vi "ByteArrayToImage.vi"(0 "CameraBytes":u8[](array[numeric]), 1 "Image":T1) -> (5 "Image Out":T1)   [LabVIEW 2019]
uses:
  <vilib>/vision/Image Controls.llb/IMAQ Image.ctl
  <vilib>/vision/NI_Vision_Development_Module.lvlib
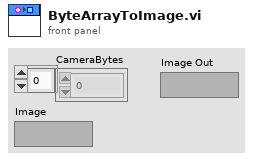
[diagram p1: front panel]
types:
  T1 = typedef "IMAQ Image.ctl" = refnum<image>
  T2 = cluster{"Red or Hue value":u8, "Green or Sat value":u8, "Blue or Luma or Val or Inten value":u8}
  T3 = cluster{"Red or Hue value":u8, "Green or Sat value":u8, "Blue or Luma or Val or Inten value":u8}[]
  T4 = cluster{"Red or Hue value":u8, "Green or Sat value":u8, "Blue or Luma or Val or Inten value":u8}[][]
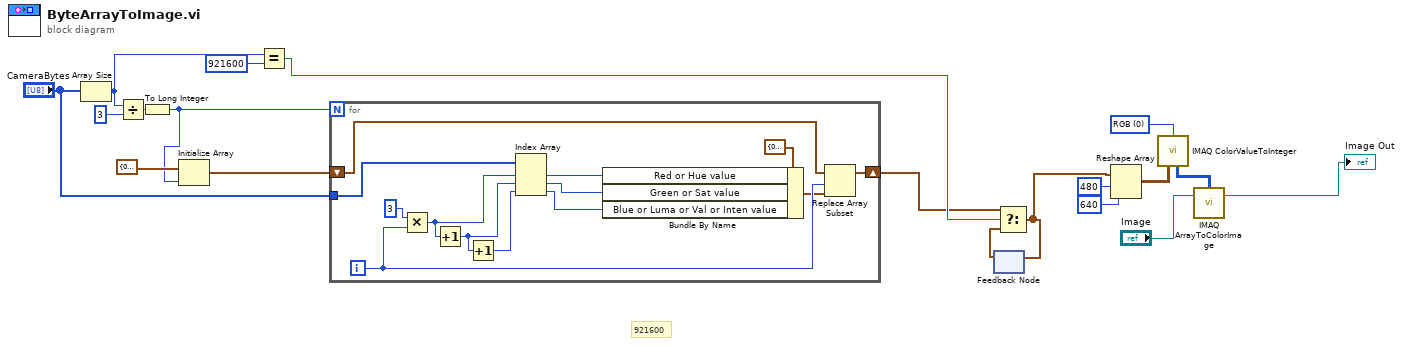
[diagram p0: block diagram]
diagram:
  w11 = u16 0 items=["RGB", "HSL", "HSV", "HSI"] ("Color Mode")
  # "921600"
  n1 = Array Size(array="CameraBytes") -> (size(s)=w1:i32)
  n2 = Divide(x=w1, y=3) -> (x/y=w17:dbl)
  n3 = To Long Integer(number=w17) -> (32bit integer=w7:i32)
  n4 = Initialize Array(T2 {"Red or Hue value"=0, "Green or Sat value"=0, "Blue or Luma or Val or Inten value"=0} ("Color Value"), w7) -> (w15:T3)
  n5 = Equal?(x=w1, y=921600) -> (x = y?=w5:bool)
  n6 = for {
    N: w7 -> [_]
    tunnel: "CameraBytes" -> [w30]
    shift-right: [w21] -> w4
    shift-left: w15 -> [w20]
    i -> [w23]
    n7 = Multiply(x=3, y=w23) -> (x*y=w26:i32)
    n8 = Increment(x=w26) -> (x+1=w25:i32)
    n9 = Increment(x=w25) -> (x+1=w24:i32)
    n10 = Index Array(array=w30, index #1=w26, index #2=w25, index #3=w24) -> (element #1=w29:u8, element #2=w28:u8, element #3=w27:u8)
    n11 = Bundle By Name(cluster=T2 {"Red or Hue value"=0, "Green or Sat value"=0, "Blue or Luma or Val or Inten value"=0} ("Color Value"), "Red or Hue value"=w29, "Green or Sat value"=w28, "Blue or Luma or Val or Inten value"=w27) -> (w22:T2)
    n12 = Replace Array Subset(array=w20, new element=w22, index=w23) -> (w21:T3)
  }
  n13 = feedback #1() -> (w2:T3)  [unwired: 1 in]
  n14 = Select(t=w4, s=w5, f=w2) -> (s? t:f=w3:T3)
  n15 = feedback-in #1(w3) -> ()
  n16 = Reshape Array(w3, 480 ("dimension size"), 640 ("dimension size")) -> (w9:T4)
  n17 = call "IMAQ ColorValueToInteger"("2D Color value array"=w9, "Color Mode"=w11) -> ("2D U32 array"=w10:u32[][])  [unwired: 3 in, 3 out]
  n18 = call "IMAQ ArrayToColorImage"("Image Pixels (U32)"=w10, "Image"="Image") -> ("Image Out"=→"Image Out":T1)  [unwired: 3 in, 1 out]
